vi "SamplingSettings.vi"(5 "Sweep Direction":bool, 7 "NLEIS Run Mode":bool caption="Test        Sweep", 8 "Peak Frequency (Hz)":dbl, 9 "Steps/Decade":dbl=10.0, 10 "Low Frequency (Hz)":dbl=1.0, 11 "High Frequency (Hz)":dbl=10000.0) -> (0 "N Samples":i32[](array[numeric]), 1 "Np Periods":i32[](array[numeric]), 2 "Freqs":dbl[](array[numeric]), 3 "Sample Rates":dbl[](array[numeric]), 4 "Frequency at \nmultiple of 60Hz":bool, 6 "Number of Frequencies":i32)   [LabVIEW 2018]
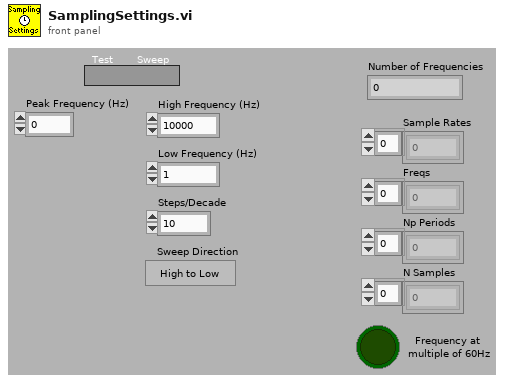
[diagram p1: front panel]
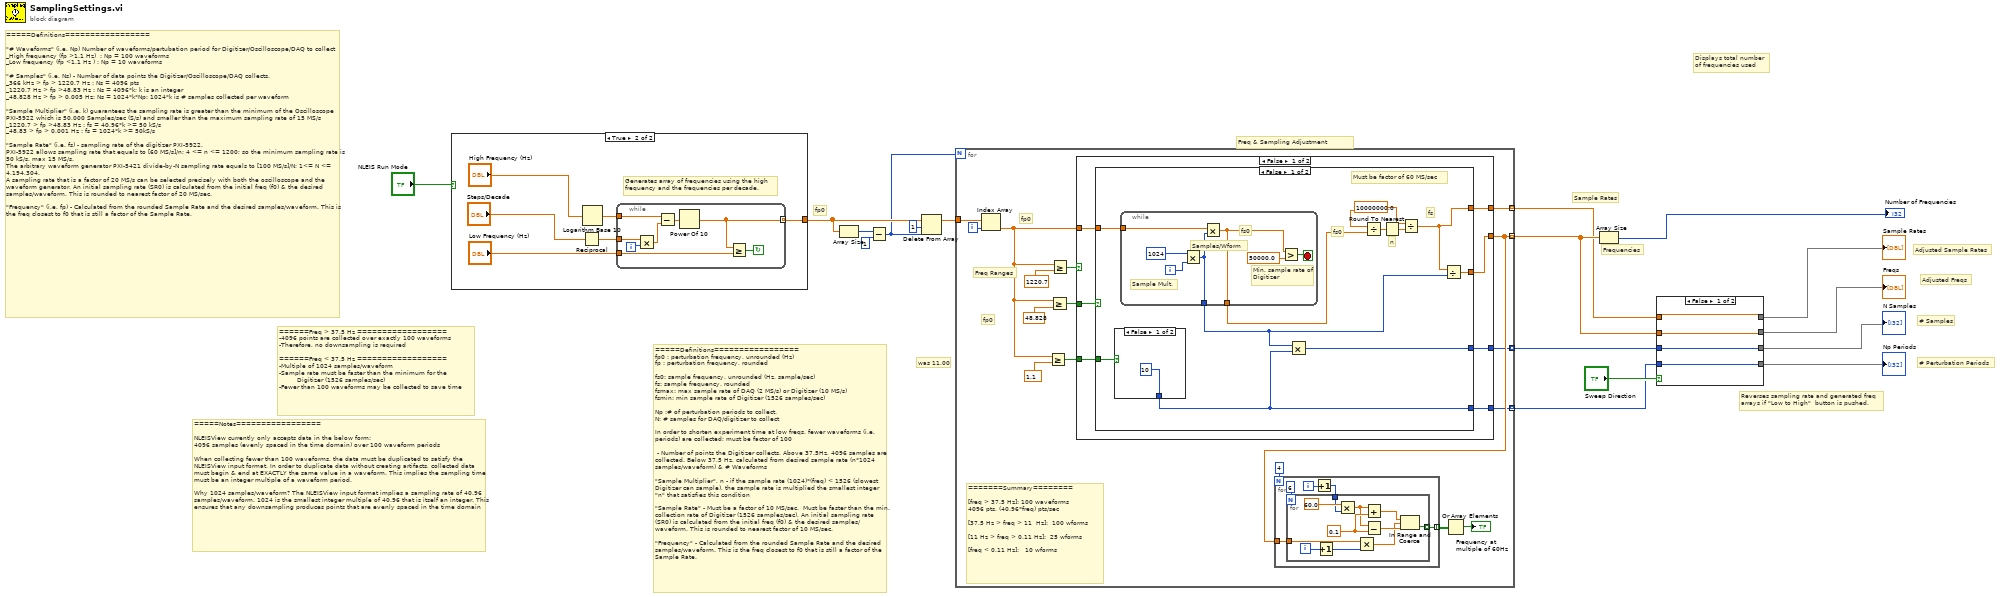
[diagram p0: block diagram]
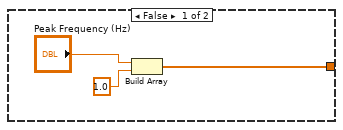
[diagram p2: hidden frame]
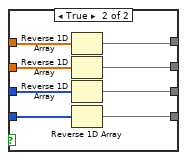
[diagram p3: hidden frame]
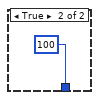
[diagram p4: hidden frame]
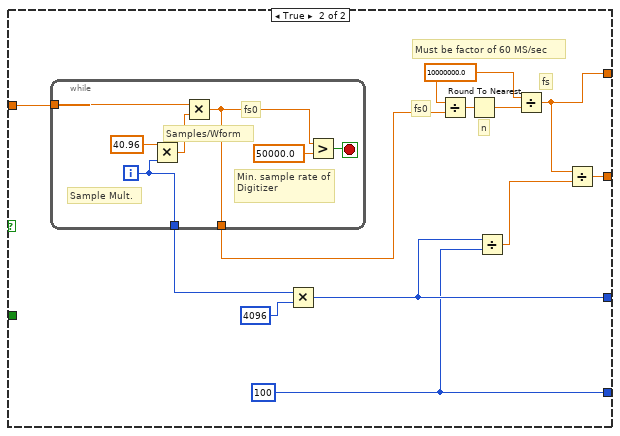
[diagram p5: hidden frame]
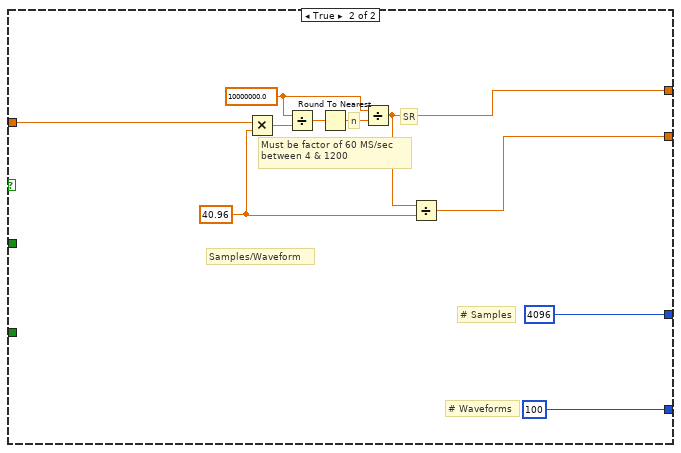
[diagram p6: hidden frame]
diagram:
  # "=====Definitions=================\nfp0 : perturbation frequency, unrounded (Hz)\nfp : perturbation frequency, rounded\n\nfs0: sample frequency, unrounded (Hz, sample/sec)\nfs: sample frequency, rounded\nfsmax: max sample rate of DAQ (2 MS/s) or Digitizer (10 MS/s)\nfsmin: min sample rate of Digitizer (1526 samples/sec)\n\nNp :# of perturbation periods to collect.\nN: # samples for DAQ/digitizer to collect\n\nIn order to shorten experiment time at low freqs, fewer waveforms (i.e. periods) are collected; must be factor of 100\n\n - Number of points the Digitizer collects. Above 37.5Hz, 4096 samples are collected. Below 37.5 Hz, calculated from desired sample rate (n*1024 samples/waveform) & # Waveforms\n\n\"Sample Multiplier\", n - if the sample rate (1024)*(freq) < 1526 (slowest Digitizer can sample), the sample rate is multiplied the smallest integer \"n\" that satisfies this condition\n\n\"Sample Rate\" - Must be a factor of 10 MS/sec.  Must be faster than the min. collection rate of Digitizer (1526 samples/sec). An initial sampling rate (SR0) is calculated from the initial freq (f0) & the desired samples/waveform. This is rounded to nearest factor of 10 MS/sec.\n\n\"Frequency\" - Calculated from the rounded Sample Rate and the desired samples/waveform. This is the freq closest to f0 that is still a factor of the Sample Rate."
  # "# Perturbation Periods"
  # "# Samples"
  # "Adjusted Freqs"
  # "Adjusted Sample Rates"
  # "was 11.00"
  # "=====Notes=================\n\nNLEISView currently only accepts data in the below form:\n4096 samples (evenly spaced in the time domain) over 100 waveform periods\n\nWhen collecting fewer than 100 waveforms, the data must be duplicated to satisfy the NLEISView input format. In order to duplicate data without creating artifacts, collected data must begin & end at EXACTLY the same value in a waveform. This implies the sampling time must be an integer multiple of a waveform period.\n\nWhy 1024 samples/waveform? The NLEISView input format implies a sampling rate of 40.96 samples/waveform. 1024 is the smallest integer multiple of 40.96 that is itself an integer. This ensures that any downsampling produces points that are evenly spaced in the time domain"
  # "=====Definitions=================\n\n\"# Waveforms\" (i.e. Np) Number of waveforms/pertubation period for Digitizer/Oscilloscope/DAQ to collect \n_High frequency (fp >1.1 Hz)  : Np = 100 waveforms\n_Low frequency (fp <1.1 Hz ) : Np = 10 waveforms\n\n\"# Samples\" (i.e. Ns) - Number of data points the Digitizer/Oscilloscope/DAQ collects. \n_366 kHz > fp > 1220.7 Hz : Ns = 4096 pts\n_1220.7 Hz > fp >48.83 Hz : Ns = 4096*k; k is an integer\n_48.828 Hz > fp > 0.005 Hz: Ns = 1024*k*Np; 1024*k is # samples collected per waveform\n\n\"Sample Multiplier\" (i.e. k) guarantees the sampling rate is greater than the minimum of the Oscilloscope PXI-5922 which is 50,000 Samples/sec (S/s) and smaller than the maximum sampling rate of 15 MS/s\n_1220.7 > fp >48.83 Hz : fs = 40.96*k >= 50 kS/s\n_48.83 > fp > 0.001 Hz : fs = 1024*k >= 50kS/s\n\n\"Sample Rate\" (i.e. fs) - sampling rate of the digitizer PXI-5922. \nPXI-5922 allows sampling rate that equals to [60 MS/s]/n; 4 <= n <= 1200; so the minimum sampling rate is 50 kS/s, max 15 MS/s. \nThe arbitrary waveform generator PXI-5421 divide-by-N sampling rate equals to [100 MS/s]/N; 1<= N <= 4,194,304.\nA sampling rate that is a factor of 20 MS/s can be selected precisely with both the oscilloscope and the waveform generator. An initial sampling rate (SR0) is calculated from the initial freq (f0) & the desired samples/waveform. This is rounded to nearest factor of 20 MS/sec.\n\n\"Frequency\" (i.e. fp) - Calculated from the rounded Sample Rate and the desired samples/waveform. This is the freq closest to f0 that is still a factor of the Sample Rate."
  # "======Freq > 37.5 Hz ==================\n-4096 points are collected over exactly 100 waveforms\n-Therefore, no downsampling is required\n\n======Freq < 37.5 Hz ==================\n-Multiple of 1024 samples/waveform\n-Sample rate must be faster than the minimum for the \n         Digitizer (1526 samples/sec)\n-Fewer than 100 waveforms may be collected to save time"
  # "Freq & Sampling Adjustment"
  # "fp0"
  # "Displays total number \nof frequencies used"
  # "Reverses sampling rate and generated freq \narrays if \"Low to High\"  button is pushed."
  # "Frequencies"
  # "Sample Rates"
  n1 = case shown="True" "NLEIS Run Mode" {
    tunnel: [w19 w23] -> w16
    frame False {
      n2 = Build Array("Peak Frequency (Hz)", 1.0) -> (w19:dbl[])
    }
    frame True {
      # "Generates array of frequencies using the high \nfrequency and the frequencies per decade."
      n3 = Reciprocal(x="Steps/Decade") -> (1/x=w24:dbl)
      n4 = Logarithm Base 10(1:"High Frequency (Hz)") -> (0:w25:dbl)
      n5 = while {
        tunnel: w25 -> [w34]
        tunnel: w24 -> [w33]
        tunnel: "Low Frequency (Hz)" -> [w29]
        tunnel: [w27] -> w23 mode=indexing
        i -> [w32]
        stop <- w28 continue-if-true
        n6 = Multiply(x=w33, y=w32) -> (x*y=w31:dbl)
        n7 = Subtract(x=w34, y=w31) -> (x-y=w30:dbl)
        n8 = Power Of 10(x=w30) -> (10^x=w27:dbl)
        n9 = Greater Or Equal?(x=w27, y=w29) -> (x >= y?=w28:bool)
      }
    }
  }
  n10 = Array Size(array=w16) -> (size(s)=w17:i32)
  n11 = Subtract(x=w17, y=1) -> (x-y=w14:i32)
  n12 = Delete From Array(array=w16, length=1 ("y"), index=w14) -> (array with subset deleted=w13:dbl[])  [unwired: 1 out]
  n13 = for {
    N: w14 -> [_]
    tunnel: w13 -> [w50]
    tunnel: [w42] -> w10 mode=indexing
    tunnel: [w43] -> w9 mode=indexing
    tunnel: [w41] -> w3 mode=indexing
    tunnel: [w40] -> w2 mode=indexing
    i -> [w49]
    # "=======Summary========\n\n[freq > 37.5 Hz]: 100 waveforms\n4096 pts, (40.96*freq) pts/sec \n\n[37.5 Hz > freq > 11  Hz]:  100 wforms\n\n[11 Hz > freq > 0.11 Hz]:  25 wforms\n\n[freq < 0.11 Hz]:   10 wforms"
    # "fp0"
    # "Freq Ranges"
    # "fp0"
    n14 = Index Array(array=w50, index=w49) -> (element=w36:dbl)
    n15 = Greater Or Equal?(x=w36, y=1.1) -> (x >= y?=w35:bool)
    n16 = Greater Or Equal?(x=w36, y=48.828) -> (x >= y?=w39:bool)
    n17 = Greater Or Equal?(x=w36, y=1220.7) -> (x >= y?=w44:bool)
    n18 = case shown="False" w44 {
      tunnel: [w55 4096 ("element")] -> w41
      tunnel: w36 -> [w57 w100]
      tunnel: [w53 w101] -> w43
      tunnel: [w52 w98] -> w42
      tunnel: [w54 100 ("element")] -> w40
      tunnel: w39 -> [w56 _]
      tunnel: w35 -> [w51 _]
      frame False {
        n19 = case shown="False" w56 {
          tunnel: w57 -> [w64 w89]
          tunnel: [w59 w82] -> w55
          tunnel: [w60 w81] -> w54
          tunnel: [w58 w79] -> w53
          tunnel: [w62 w78] -> w52
          tunnel: w51 -> [w63 _]
          frame False {
            w65 = 10000000.0 ("y")
            # "Must be factor of 60 MS/sec"
            # "fs0"
            # "fs"
            # "n"
            n20 = case shown="False" w63 {
              tunnel: [10 100] -> w60
              frame False {
              }
              frame True {
              }
            }
            n21 = while {
              tunnel: [w75] -> w68
              tunnel: [w71] -> w61
              tunnel: w64 -> [w72]
              i -> [w74]
              stop <- w76 stop-if-true
              # "Sample Mult."
              # "Samples/Wform"
              # "fs0"
              # "Min. sample rate of Digitizer"
              n22 = Multiply(x=1024, y=w74) -> (x*y=w71:i32)
              n23 = Multiply(x=w72, y=w71) -> (x*y=w75:dbl)
              n24 = Greater?(x=w75, y=50000.0) -> (0:w76:bool)
            }
            n25 = Multiply(x=w61, y=w60) -> (x*y=w59:i32)
            n26 = Divide(x=w65, y=w68) -> (x/y=w66:dbl)
            n27 = Round To Nearest(number=w66) -> (nearest integer value=w67:dbl)
            n28 = Divide(x=w65, y=w67) -> (x/y=w58:dbl)
            n29 = Divide(x=w58, y=w61) -> (x/y=w62:dbl)
          }
          frame True {
            w85 = 10000000.0 ("y")
            w81 = 100
            # "Must be factor of 60 MS/sec"
            # "fs0"
            # "fs"
            # "n"
            n30 = while {
              tunnel: w89 -> [w94]
              tunnel: [w93] -> w83
              tunnel: [w90] -> w88
              i -> [w90]
              stop <- w95 stop-if-true
              # "Sample Mult."
              # "Samples/Wform"
              # "fs0"
              # "Min. sample rate of Digitizer"
              n31 = Multiply(x=40.96 ("y"), y=w90) -> (x*y=w92:dbl)
              n32 = Multiply(x=w94, y=w92) -> (x*y=w93:dbl)
              n33 = Greater?(x=w93, y=50000.0) -> (0:w95:bool)
            }
            n34 = Multiply(x=w88, y=4096) -> (x*y=w82:i32)
            n35 = Divide(x=w85, y=w83) -> (x/y=w86:dbl)
            n36 = Round To Nearest(number=w86) -> (nearest integer value=w84:dbl)
            n37 = Divide(x=w82, y=w81) -> (x/y=w80:dbl)
            n38 = Divide(x=w85, y=w84) -> (x/y=w79:dbl)
            n39 = Divide(x=w79, y=w80) -> (x/y=w78:dbl)
          }
        }
      }
      frame True {
        w99 = 40.96 ("y")
        w103 = 10000000.0 ("y")
        # "Must be factor of 60 MS/sec\nbetween 4 & 1200"
        # "# Waveforms"
        # "Samples/Waveform"
        # "SR"
        # "n"
        # "# Samples"
        n40 = Multiply(x=w100, y=w99) -> (x*y=w105:dbl)
        n41 = Divide(x=w103, y=w105) -> (x/y=w104:dbl)
        n42 = Round To Nearest(number=w104) -> (nearest integer value=w102:dbl)
        n43 = Divide(x=w103, y=w102) -> (x/y=w101:dbl)
        n44 = Divide(x=w101, y=w99) -> (x/y=w98:dbl)
      }
    }
    n45 = for {
      N: 4 -> [_]
      tunnel: [w108] -> w46 mode=indexing
      tunnel: w42 -> [w107]
      i -> [w111]
      n46 = Increment(x=w111) -> (x+1=w110:i32)
      n47 = for {
        N: 6 -> [_]
        tunnel: w110 -> [w115]
        tunnel: [w113] -> w108 mode=indexing
        tunnel: w107 -> [w112]
        i -> [w117]
        w122 = 0.1
        n48 = Increment(x=w117) -> (x+1=w116:i32)
        n49 = Multiply(x=60.0, y=w115) -> (x*y=w119:dbl)
        n50 = Multiply(x=w112, y=w116) -> (x*y=w114:dbl)
        n51 = Add(x=w119, y=w122) -> (x+y=w121:dbl)
        n52 = Subtract(x=w119, y=w122) -> (x-y=w120:dbl)
        n53 = In Range and Coerce(upper limit=w121, x=w114, lower limit=w120) -> (In Range?=w113:bool)  [unwired: 1 out]
      }
    }
    n54 = Or Array Elements(Boolean array=w46) -> (logical OR=→"Frequency at \nmultiple of 60Hz":bool)
  }
  n55 = Array Size(array=w10) -> (size(s)=→"Number of Frequencies":i32)
  n56 = case shown="False" "Sweep Direction" {
    tunnel: w10 -> [w125 w132]
    tunnel: w9 -> [w126 w134]
    tunnel: [w126 w133] -> w8
    tunnel: [w125 w131] -> w7
    tunnel: [w124 w129] -> w4
    tunnel: w3 -> [w124 w130]
    tunnel: w2 -> [w123 w128]
    tunnel: [w123 w127] -> w1
    frame False {
    }
    frame True {
      n57 = Reverse 1D Array(array=w134) -> (reversed array=w133:dbl[])
      n58 = Reverse 1D Array(array=w132) -> (reversed array=w131:dbl[])
      n59 = Reverse 1D Array(array=w130) -> (reversed array=w129:i32[])
      n60 = Reverse 1D Array(array=w128) -> (reversed array=w127:i32[])
    }
  }
  "Sample Rates" <- w8
  "Freqs" <- w7
  "N Samples" <- w4
  "Np Periods" <- w1
